vi "RGB32 Smooth.vi"(11 "image":u32[][](array[numeric])) -> (3 "Smoothed":u32[][](array[numeric]))   [LabVIEW 2017]
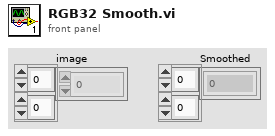
[diagram p1: front panel]
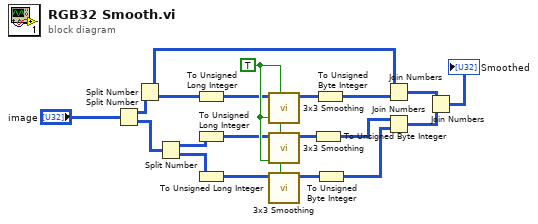
[diagram p0: block diagram]
diagram:
  w18 = TRUE ("Enable")
  n1 = Split Number(x="image") -> (hi(x)=w13:u16[][], lo(x)=w12:u16[][])
  n2 = Split Number(x=w13) -> (hi(x)=w14:u8[][], lo(x)=w19:u8[][])
  n3 = Split Number(x=w12) -> (hi(x)=w11:u8[][], lo(x)=w10:u8[][])
  n4 = To Unsigned Long Integer(number=w19) -> (unsigned 32bit integer=w17:u32[][])
  n5 = To Unsigned Long Integer(number=w11) -> (unsigned 32bit integer=w16:u32[][])
  n6 = To Unsigned Long Integer(number=w10) -> (unsigned 32bit integer=w15:u32[][])
  n7 = call "3x3 Smoothing.vi"("Enable"=w18, "Image"=w17) -> ("Smoothed"=w9:u32[][])  [unwired: 9 in]
  n8 = call "3x3 Smoothing.vi"("Enable"=w18, "Image"=w16) -> ("Smoothed"=w8:u32[][])  [unwired: 9 in]
  n9 = call "3x3 Smoothing.vi"("Enable"=w18, "Image"=w15) -> ("Smoothed"=w7:u32[][])  [unwired: 9 in]
  n10 = To Unsigned Byte Integer(number=w8) -> (unsigned 8bit integer=w3:u8[][])
  n11 = To Unsigned Byte Integer(number=w9) -> (unsigned 8bit integer=w4:u8[][])
  n12 = To Unsigned Byte Integer(number=w7) -> (unsigned 8bit integer=w2:u8[][])
  n13 = Join Numbers(hi=w14, lo=w4) -> ((hi.lo)=w6:u16[][])
  n14 = Join Numbers(hi=w3, lo=w2) -> ((hi.lo)=w5:u16[][])
  n15 = Join Numbers(hi=w6, lo=w5) -> ((hi.lo)=→"Smoothed":u32[][])
